vi "CmdExe.Merge StdOut and StdError.vi"(4 "PASS Result Code":i32, 6 "Result Code":i32, 8 "error in":errorcluster, 9 "Error Key Phrases":string[](array[string]), 10 "StdErr":string, 11 "StdOut":string) -> (0 "error out":errorcluster, 3 "Std Out + Error":string)   [LabVIEW 2018]
uses:
  Errors/Error.Error Code List.ctl
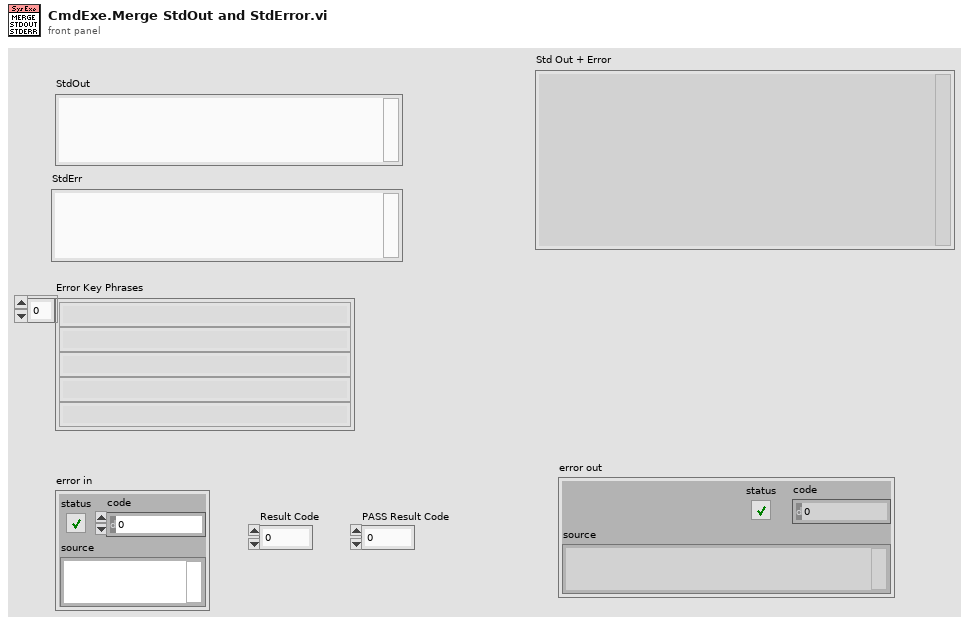
[diagram p1: front panel]
types:
  T1 = typedef "Error.Error Code List.ctl" = i32
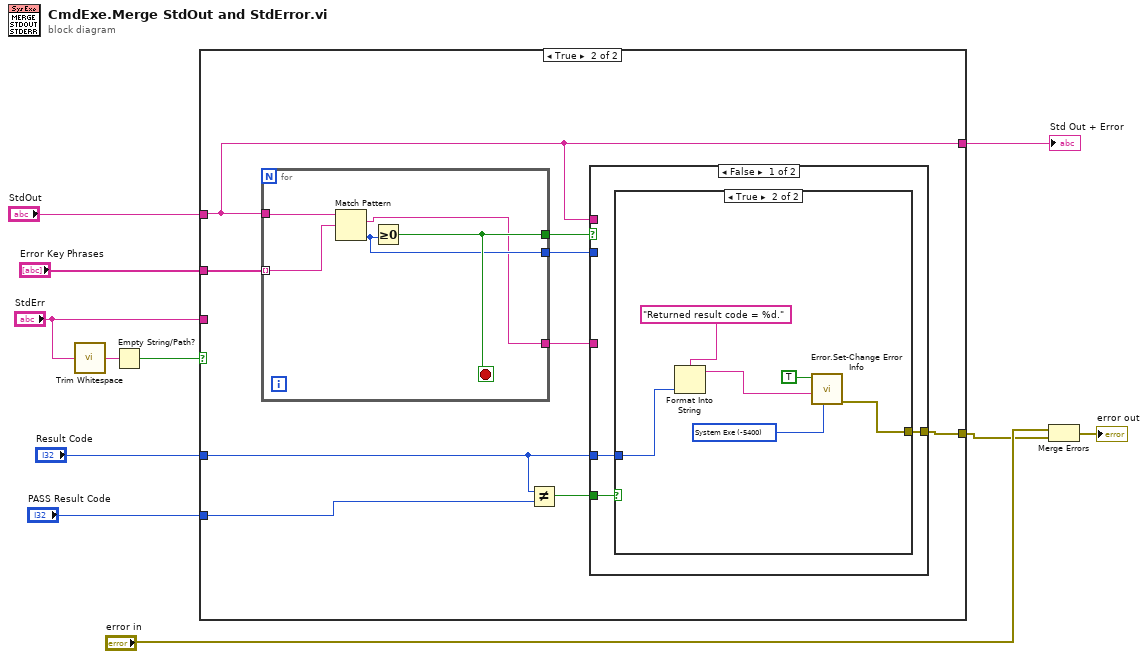
[diagram p0: block diagram]
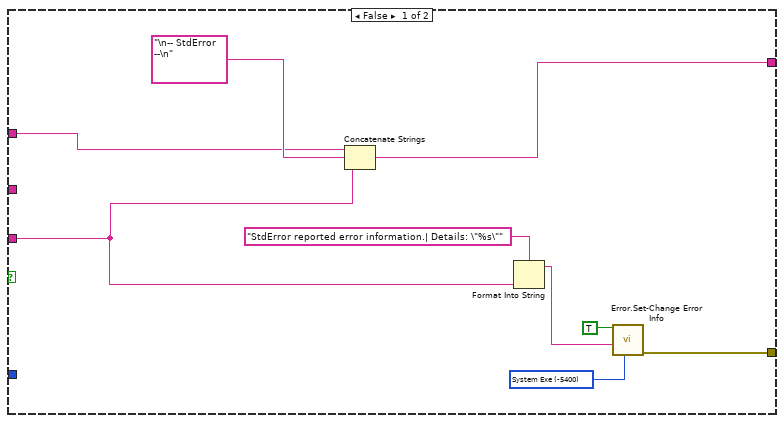
[diagram p2: hidden frame]
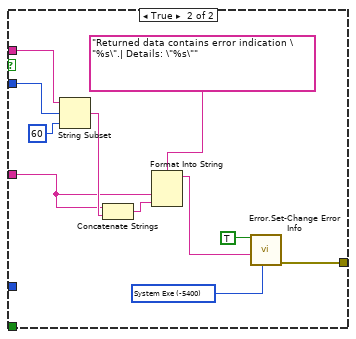
[diagram p4: hidden frame]
diagram:
  n1 = call <vilib>:"Trim Whitespace.vi"("string"="StdErr") -> ("trimmed string"=w10:string)  [unwired: 1 in]
  n2 = Empty String/Path?(string/path=w10) -> (empty?=w9:bool)
  n3 = case shown="True" w9 {
    tunnel: "StdErr" -> [w12 _]
    tunnel: "StdOut" -> [w14 w24]
    tunnel: "Error Key Phrases" -> [_ w26]
    tunnel: [w16 w27] -> w3
    tunnel: [w13 w24] -> w11
    tunnel: "Result Code" -> [_ w23]
    tunnel: "PASS Result Code" -> [_ w22]
    frame False {
      w18 = T1 -5400 items=["No Error"=0, "Abort"=-2, "Misc"=-5000, "Fixture Error"=-5100, "File IO - General"=-5200, "FIle IO - Config Error"=-5201, "Instrument - General"=-5300, "Instrument - Serial Com"=-5301, "Instrument - Camera"=-5302, "Instrument - PS"=-5303, "Instrument - Oscilloscope"=-5304, "Instrument - Function Gen"=-5305, "Instrument - Load"=-5306, "Instrument - Meter"=-5307, "Instrument - Power Control"=-5308, "Instrument - Motion"=-5309, "Instrument - RF"=-5310, "System Exe"=-5400, "Image Processing"=-5500, "Communication"=-5600, "Script - Syntax Error"=-6000, "Script - Invalid Name or Param"=-6100, "Script - Timeout"=-6200, "Invalid Data"=-6300] ("Std Code")
      n4 = Concatenate Strings(w14, "\n-- StdError --\n", w12) -> (w13:string)
      n5 = Format Into String(format string="StdError reported error information.| Details: \"%s\"", w12) -> (resulting string=w17:string)  [unwired: 2 in, 1 out]
      n6 = call "Error.Set-Change Error Info.vi"("Std Code"=w18, "Description"=w17, "Set Error"=TRUE) -> ("error out"=w16:errorcluster)  [unwired: 8 in]
    }
    frame True {
      n7 = for {
        tunnel: w24 -> [w54]
        tunnel: [w51] -> w28
        tunnel: [w53] -> w29
        tunnel: w26 -> [w50] mode=indexing
        tunnel: [w52] -> w25
        stop <- w53 stop-if-true
        n8 = Match Pattern(string=w54, regular expression=w50) -> (match substring=w51:string, offset past match=w52:i32)  [unwired: 1 in, 2 out]
        n9 = Greater Or Equal To 0?(x=w52) -> (x >= 0?=w53:bool)
      }
      n10 = Not Equal?(x=w23, y=w22) -> (x != y?=w21:bool)
      n11 = case shown="False" w29 {
        tunnel: w28 -> [_ w39]
        tunnel: [w30 w45] -> w27
        tunnel: w25 -> [_ w44]
        tunnel: w24 -> [_ w42]
        tunnel: w23 -> [w32 _]
        tunnel: w21 -> [w31 _]
        frame False {
          n12 = case shown="True" w31 {
            tunnel: w32 -> [_ w34]
            tunnel: [_ w33] -> w30
            frame False {
            }
            frame True {
              w38 = T1 -5400 items=["No Error"=0, "Abort"=-2, "Misc"=-5000, "Fixture Error"=-5100, "File IO - General"=-5200, "FIle IO - Config Error"=-5201, "Instrument - General"=-5300, "Instrument - Serial Com"=-5301, "Instrument - Camera"=-5302, "Instrument - PS"=-5303, "Instrument - Oscilloscope"=-5304, "Instrument - Function Gen"=-5305, "Instrument - Load"=-5306, "Instrument - Meter"=-5307, "Instrument - Power Control"=-5308, "Instrument - Motion"=-5309, "Instrument - RF"=-5310, "System Exe"=-5400, "Image Processing"=-5500, "Communication"=-5600, "Script - Syntax Error"=-6000, "Script - Invalid Name or Param"=-6100, "Script - Timeout"=-6200, "Invalid Data"=-6300] ("Std Code")
              n13 = Format Into String(format string="Returned result code = %d.", w34) -> (resulting string=w35:string)  [unwired: 2 in, 1 out]
              n14 = call "Error.Set-Change Error Info.vi"("Std Code"=w38, "Description"=w35, "Set Error"=TRUE) -> ("error out"=w33:errorcluster)  [unwired: 8 in]
            }
          }
        }
        frame True {
          w47 = T1 -5400 items=["No Error"=0, "Abort"=-2, "Misc"=-5000, "Fixture Error"=-5100, "File IO - General"=-5200, "FIle IO - Config Error"=-5201, "Instrument - General"=-5300, "Instrument - Serial Com"=-5301, "Instrument - Camera"=-5302, "Instrument - PS"=-5303, "Instrument - Oscilloscope"=-5304, "Instrument - Function Gen"=-5305, "Instrument - Load"=-5306, "Instrument - Meter"=-5307, "Instrument - Power Control"=-5308, "Instrument - Motion"=-5309, "Instrument - RF"=-5310, "System Exe"=-5400, "Image Processing"=-5500, "Communication"=-5600, "Script - Syntax Error"=-6000, "Script - Invalid Name or Param"=-6100, "Script - Timeout"=-6200, "Invalid Data"=-6300] ("Std Code")
          n15 = String Subset(string=w42, offset (0)=w44, length (rest)=60 ("length (rest)")) -> (substring=w40:string)
          n16 = Concatenate Strings(w39, w40) -> (w41:string)
          n17 = Format Into String(format string="Returned data contains error indication \"%s\".| Details: \"%s\"", w39, w41) -> (resulting string=w46:string)  [unwired: 2 in, 1 out]
          n18 = call "Error.Set-Change Error Info.vi"("Std Code"=w47, "Description"=w46, "Set Error"=TRUE) -> ("error out"=w45:errorcluster)  [unwired: 8 in]
        }
      }
    }
  }
  "Std Out + Error" <- w11
  n19 = Merge Errors("error in", w3) -> (→"error out":errorcluster)
